vi "LJUD UE9RAW WatchdogConfig.vi"(4 "DAC Parameters":T1={"DAC0"=0, "DAC1"=0, "Enable DACs"=TRUE}, 6 "DIO Parameters":cluster{"DIOConfigA":u8, "DIOConfigB":u8}, 7 "Comm Settings":T2={"Open LabJack "=TRUE, "Use USB"=TRUE, "IP Address"="192.168.1.209", "PortA"=52360, "PortB"=0}, 8 "error in (no error)":errorcluster, 9 "TimeoutPeriod":u16=10, 10 "WatchdogOptions":u8, 11 "Handle In":i32) -> (0 "error out":errorcluster, 3 "Handle Out":i32)   [LabVIEW 2021]
panel:
  # "Bit 6:  Reset Comm\nBit 5:  Reset Control\nBit 4:  Update Digital I/O B\nBit 3:  Update Digital I/O A\nBit 1:  Update DAC1 on Timeout\nBit 0:  Update DAC0 on Timeout"
  # "~Seconds"
  # "0-4095"
  # "Bit 7:  State\nBit 4-0:  Digital I/O #"
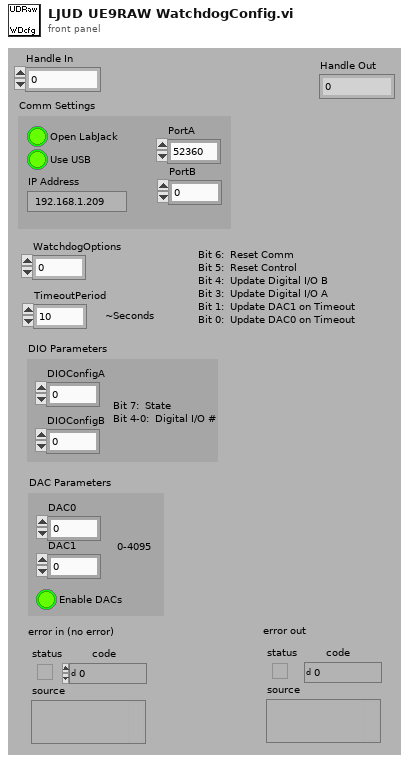
[diagram p1: front panel]
types:
  T1 = cluster{"DAC0":u16, "DAC1":u16, "Enable DACs":bool}
  T2 = cluster{"Open LabJack ":bool, "Use USB":bool, "IP Address":string, "PortA":u16, "PortB":u16}
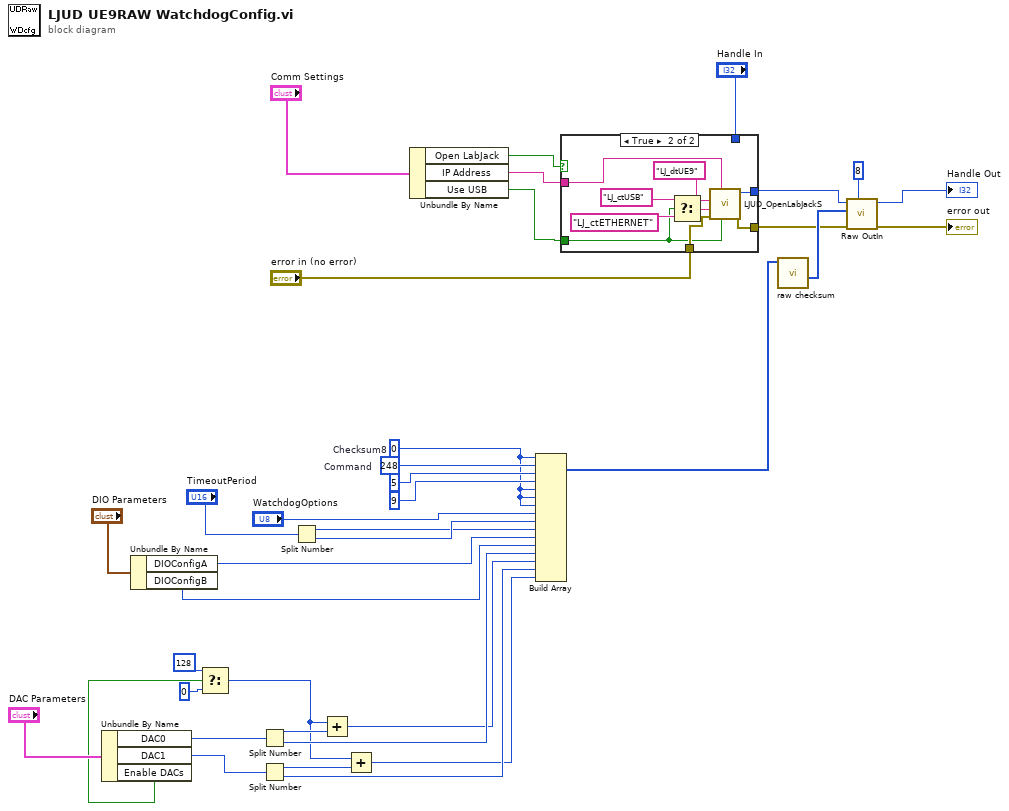
[diagram p0: block diagram]
diagram:
  w26 = u8 0  # Checksum8
  w37 = u8 248  # Command
  n1 = Unbundle By Name("DAC Parameters") -> ("DAC0"=w5:u16, "DAC1"=w4:u16, "Enable DACs"=w6:bool)
  n2 = Unbundle By Name("DIO Parameters") -> ("DIOConfigA"=w2:u8, "DIOConfigB"=w1:u8)
  n3 = Select(t=u8 128 ("x"), s=w6, f=u8 0 ("x")) -> (s? t:f=w21:u8)
  n4 = Split Number(x=w5) -> (hi(x)=w30:u8, lo(x)=w25:u8)
  n5 = Split Number(x=w4) -> (hi(x)=w29:u8, lo(x)=w23:u8)
  n6 = Split Number(x="TimeoutPeriod") -> (hi(x)=w31:u8, lo(x)=w32:u8)
  n7 = Add(x=w21, y=w30) -> (x+y=w24:u8)
  n8 = Add(x=w21, y=w29) -> (x+y=w22:u8)
  n9 = Unbundle By Name("Comm Settings") -> ("Open LabJack"=w18:bool, "IP Address"=w17:string, "Use USB"=w16:bool)
  n10 = Build Array(w26, w37, u8 5, u8 9, w26, w26, w26, "WatchdogOptions", w32, w31, w2, w1, w25, w24, w23, w22) -> (w13:u8[])
  n11 = case shown="True" w18 {
    tunnel: w17 -> [_ w42]
    tunnel: "error in (no error)" -> [w39 w46]
    tunnel: [w39 w45] -> w15
    tunnel: [w38 w43] -> w14
    tunnel: w16 -> [_ w44]
    tunnel: "Handle In" -> [w38 _]
    frame False {
    }
    frame True {
      n12 = Select(t="LJ_ctUSB" ("ConnectionType"), s=w44, f="LJ_ctETHERNET" ("ConnectionType")) -> (s? t:f=w40:string)
      n13 = call "LJUD_OpenLabJackS.vi"("FirstFound"=w44, "Address"=w42, "error in"=w46, "ConnectionType"=w40, "DeviceType"="LJ_dtUE9") -> ("error out"=w45:errorcluster, "Handle"=w43:i32)  [unwired: 4 in, 1 out]
    }
  }
  n14 = call "raw checksum.vi"("Array"=w13) -> ("Array Output"=w20:u8[])  [unwired: 3 in, 7 out]
  n15 = call "Raw OutIn.vi"("# of bytes to read in"=8 ("# of bytes to read"), "error in"=w15, "Raw Out"=w20, "Handle In"=w14) -> ("error out"=→"error out":errorcluster, "Handle Out"=→"Handle Out":i32)  [unwired: 4 in, 2 out]
